vi "spring.vi"(7 "action (set itemstrings)":T1=enum."set itemstrings", 8 "error in (no error)":errorcluster, 9 "indentation/item symbols/colors in":i32[](array[numeric]), 10 "item strings in":string[][](array[string]), 11 "tree RefNum in":refnum<vi>) -> (0 "error out":errorcluster, 1 "item symbols/colors out":i32[](array[numeric]), 2 "item strings out":string[][](array[string]), 3 "dup tree RefNum":refnum<vi>)   [LabVIEW 2014]
uses:
  <userlib>/MSC-Tree/SW Code/Tree -string-/sub VIs/spring action.ctl
  <userlib>/MSC-Tree/SW Code/Tree -string-/sub VIs/spring - node data.ctl
panel:
  # "If you get error 16,\nthe number of columns\nin the input and tree\ndoes not match."
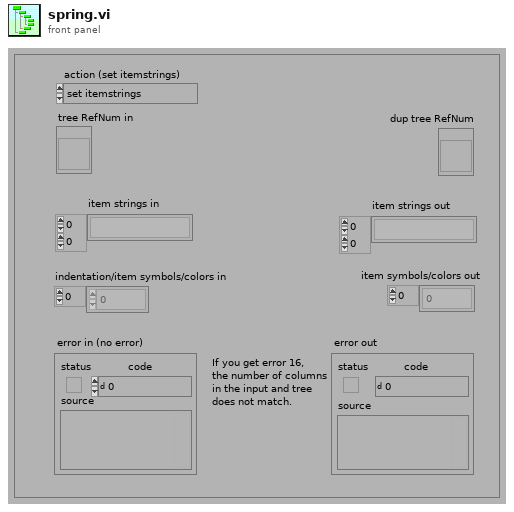
[diagram p1: front panel]
types:
  T1 = typedef "spring action.ctl" = enum16{"_init", "_add tree", "set itemstrings", "set fg colors", "set bg colors", "set symbols", "get tags", "get itemstrings", "get fg colors", "get bg colors", "get symbols", "empty tree", "update from tree"}
  T2 = typedef "spring - node data.ctl" = cluster{"tag":string, "indentation":i32, "itemstrings":string[], "fg color":i32, "bg color":i32, "symbol":i32}
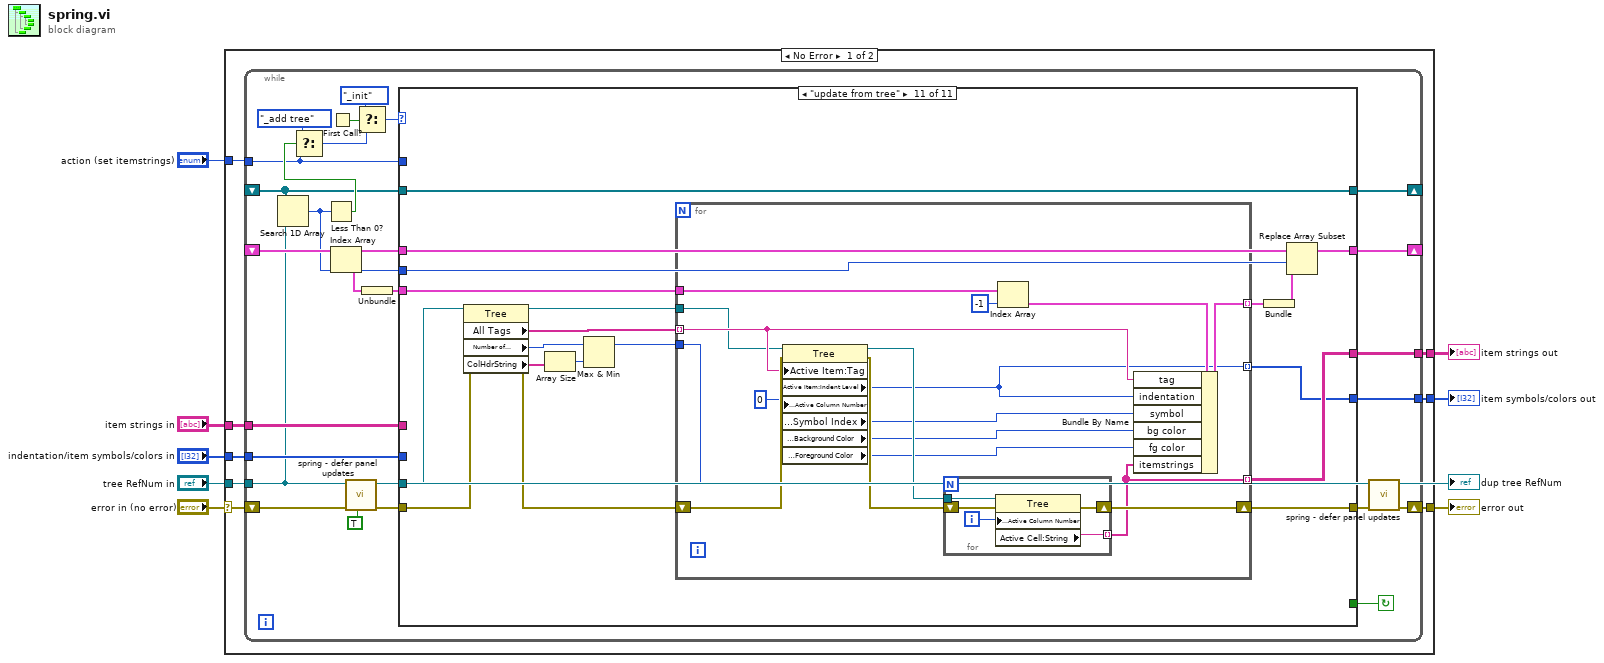
[diagram p0: block diagram]
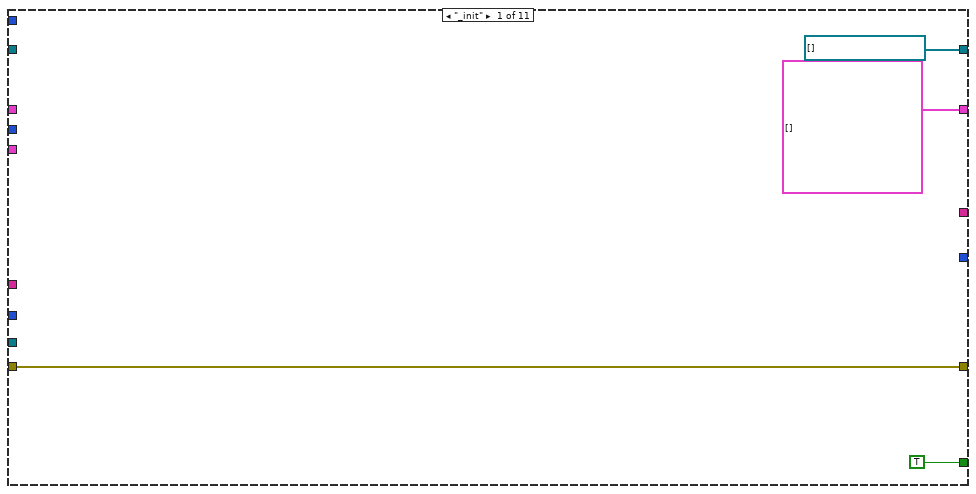
[diagram p2: hidden frame]
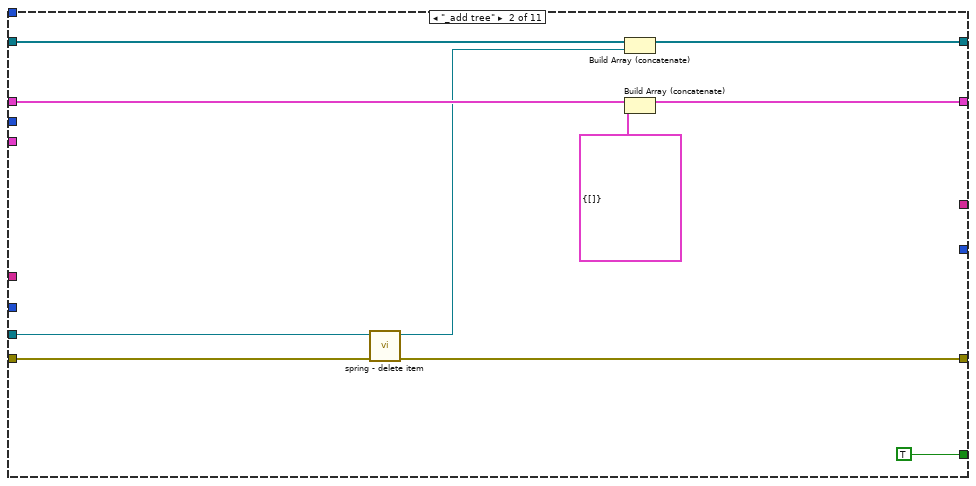
[diagram p3: hidden frame]
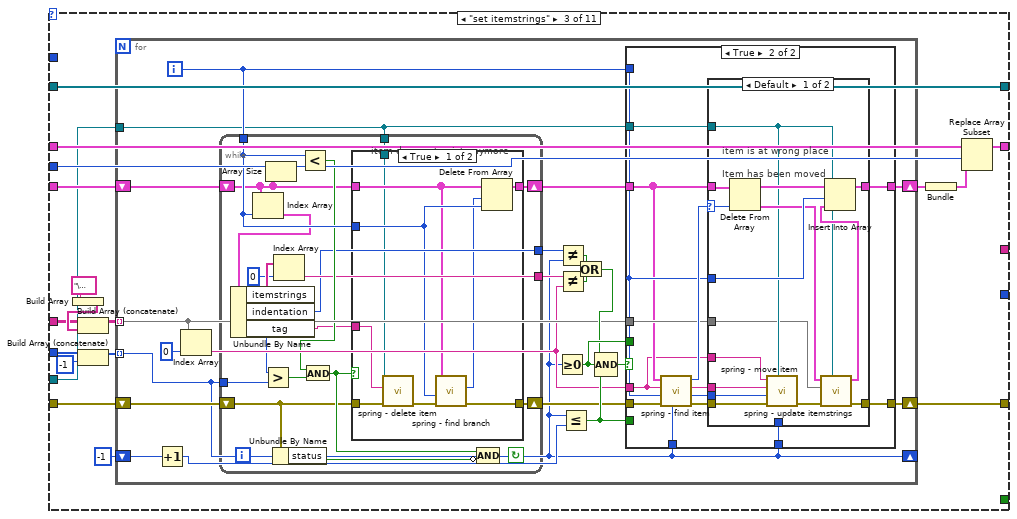
[diagram p4: hidden frame]
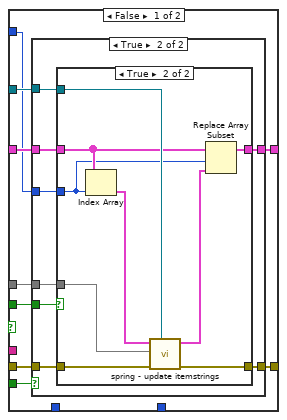
[diagram p6: hidden frame]
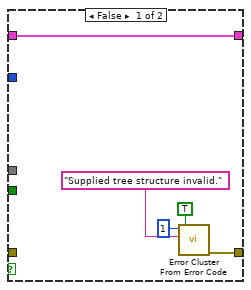
[diagram p7: hidden frame]
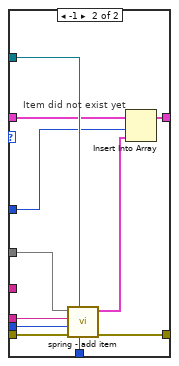
[diagram p9: hidden frame]
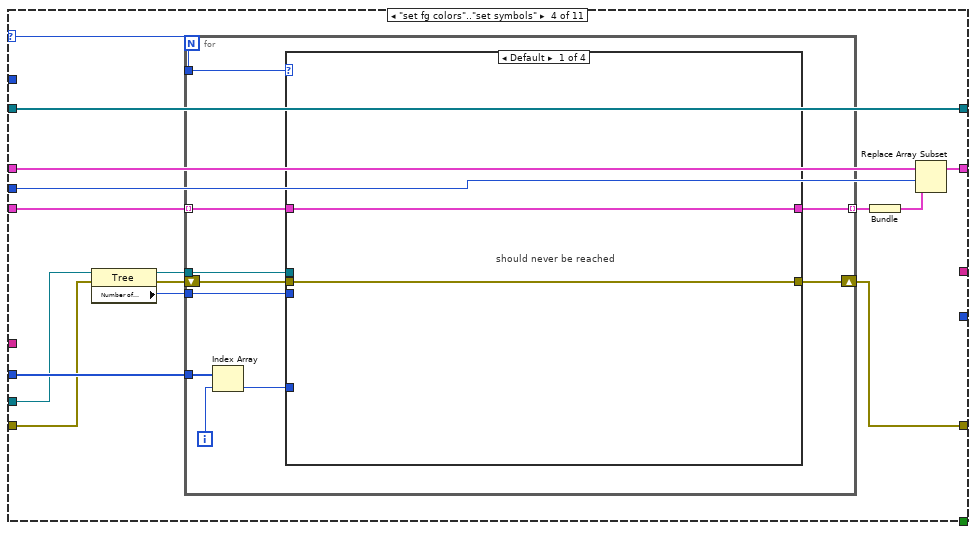
[diagram p10: hidden frame]
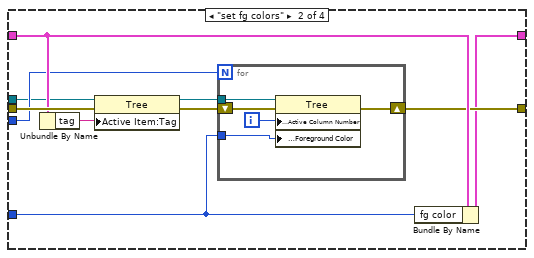
[diagram p11: hidden frame]
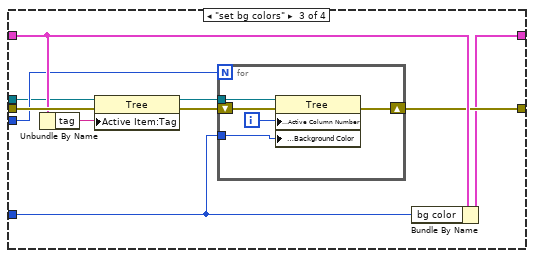
[diagram p12: hidden frame]
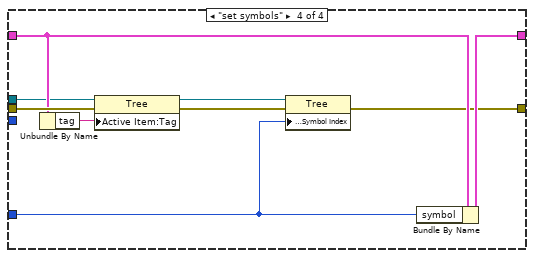
[diagram p13: hidden frame]
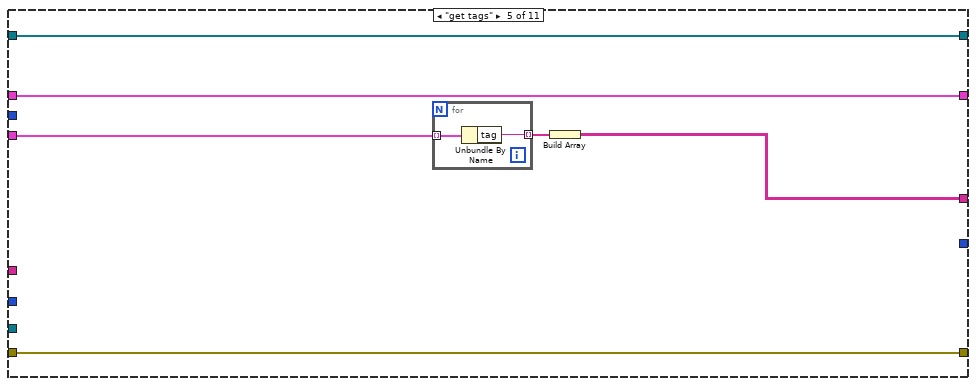
[diagram p14: hidden frame]
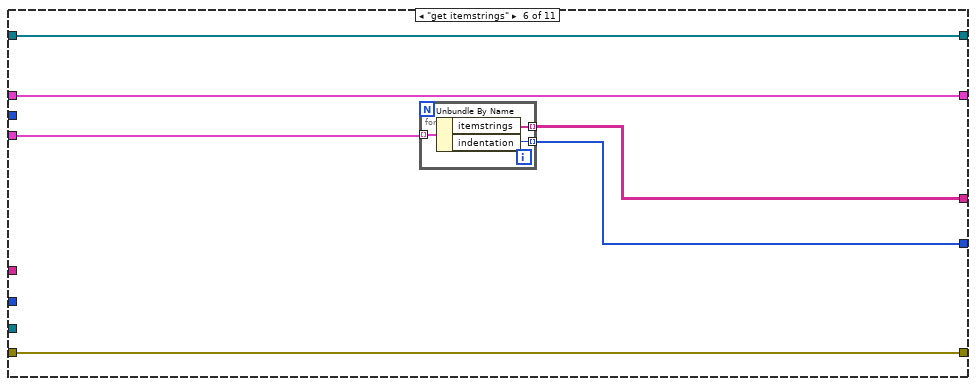
[diagram p15: hidden frame]
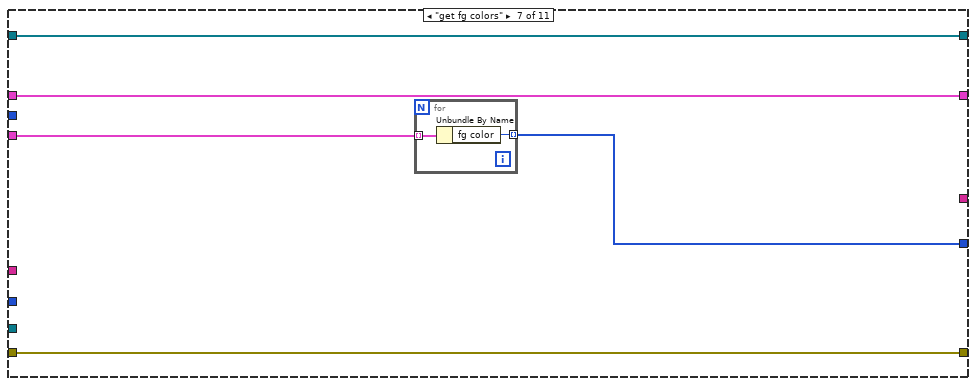
[diagram p16: hidden frame]
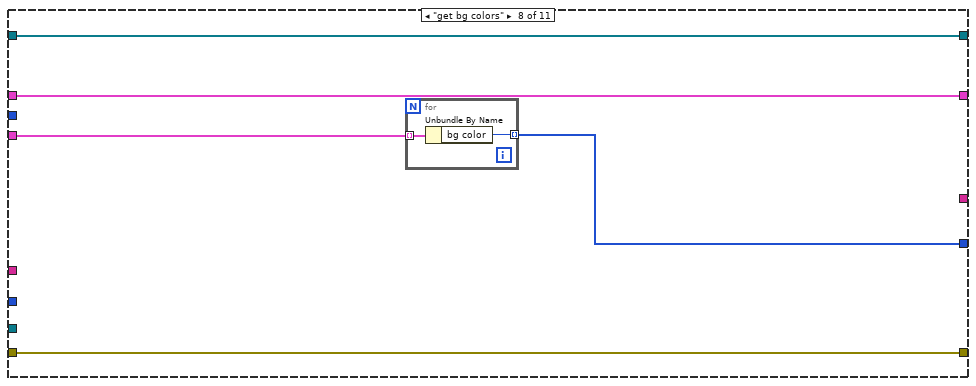
[diagram p17: hidden frame]
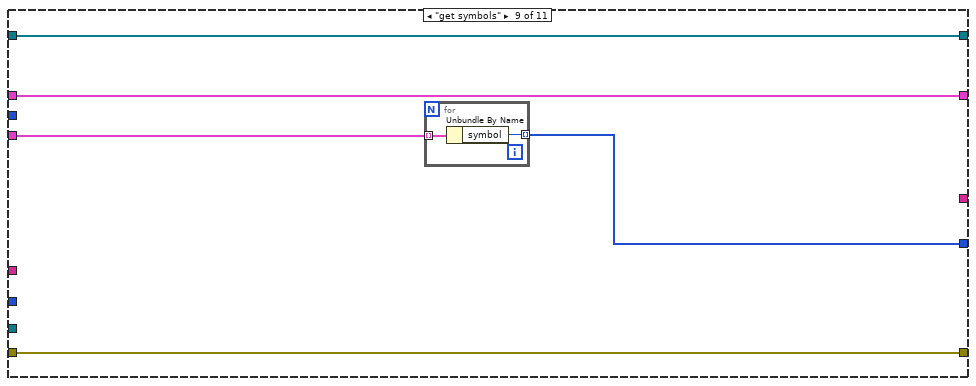
[diagram p18: hidden frame]
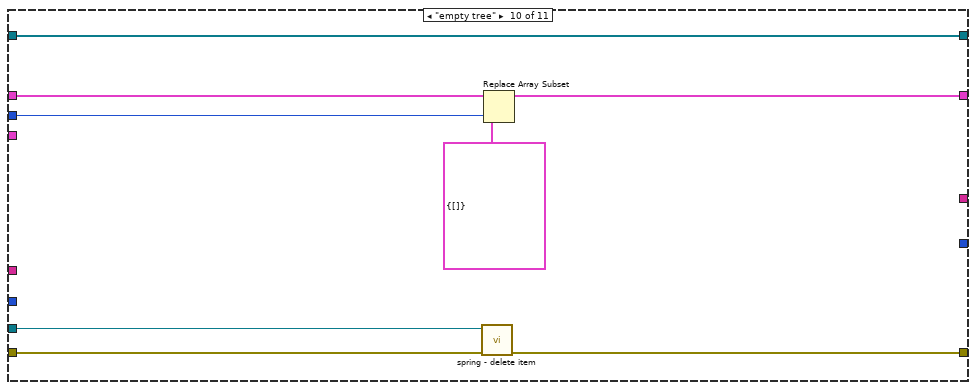
[diagram p19: hidden frame]
diagram:
  n1 = case shown="No Error" "error in (no error)" {
    selector: "error in (no error)" -> [w15 w353]
    tunnel: "tree RefNum in" -> [w16 _]
    tunnel: [w14 w353] -> w4
    tunnel: "item strings in" -> [w13 _]
    tunnel: "action (set itemstrings)" -> [w12 _]
    tunnel: [w11 _] -> w3
    tunnel: "indentation/item symbols/colors in" -> [w10 _]
    tunnel: [w9 _] -> w6
    frame No Error {
      n2 = while {
        tunnel: w16 -> [w19]
        shift-right: [w37] -> _
        shift-left: _ -> [w36]
        shift-right: [w23] -> w14
        shift-left: w15 -> [w22]
        tunnel: w13 -> [w35]
        shift-right: [w33] -> _
        shift-left: _ -> [w32]
        tunnel: [w29] -> w11
        tunnel: w10 -> [w26]
        tunnel: [w25] -> w9
        tunnel: w12 -> [w17]
        stop <- w34 continue-if-true
        n3 = Search 1D Array(1D array=w36, element=w19) -> (index of element=w30:i32)  [unwired: 1 out]
        n4 = Less Than 0?(x=w30) -> (x < 0?=w40:bool)
        n5 = Select(t=spring_action."_add tree" ("action"), s=w40, f=w17) -> (s? t:f=w42:T1)
        n6 = First Call?() -> (First Call?: T/F=w41:bool)
        n7 = Index Array(array=w32, index=w30) -> (element=w28:cluster{T2[]})
        n8 = call <userlib>:"spring - defer panel updates.vi"("defer panelUpdates (F)"=TRUE ("enable panel updates"), "error in (no error)"=w22, "RefNum in"=w19) -> ("error out"=w20:errorcluster, "dup RefNum"=w18:refnum<vi>)  [unwired: 2 in, 5 out]
        n9 = Select(t=spring_action."_init" ("action"), s=w41, f=w42) -> (s? t:f=w39:T1)
        n10 = Unbundle(w28) -> (w27:T2[])
        n11 = case shown="\"update from tree\"" w39 {
          selector: w39 -> [_ _ _ w206 _ _ _ _ _ _ _]
          tunnel: w20 -> [w45 w51 w58 w202 w269 w274 w285 w292 w299 w309 w321]
          tunnel: [w45 w50 w59 w200 w269 w274 w285 w292 w299 w308 w322] -> w24
          tunnel: w17 -> [_ _ _ _ _ _ _ _ _ _ _]
          tunnel: [refnum<vi>[] [] ("initialized array") w56 w74 w214 w270 w278 w286 w293 w300 w305 w330] -> w37
          tunnel: w36 -> [_ w55 w74 w214 w270 w278 w286 w293 w300 w305 w330]
          tunnel: w35 -> [_ _ w60 _ _ _ _ _ _ _ _]
          tunnel: [TRUE TRUE _ _ _ _ _ _ _ _ _] -> w34
          tunnel: w30 -> [_ _ w71 w211 _ _ _ _ _ w306 w328]
          tunnel: w32 -> [_ w52 w72 w212 w271 w279 w287 w294 w301 w311 w329]
          tunnel: [cluster{T2[]}[] [] ("initialized array") w54 w73 w213 w271 w279 w287 w294 w301 w310 w319] -> w33
          tunnel: [_ _ _ _ w267 w276 _ _ _ _ w324] -> w29
          tunnel: w27 -> [_ _ w65 w209 w268 w277 w284 w291 w298 _ w325]
          tunnel: w26 -> [_ _ w63 w203 _ _ _ _ _ _ _]
          tunnel: [_ _ _ _ _ w275 w283 w290 w297 _ w323] -> w25
          tunnel: w18 -> [_ w48 w57 w201 _ _ _ _ _ w307 w320]
          frame "_init" {
          }
          frame "_add tree" {
            n12 = call <userlib>:"spring - delete item.vi"("error in (no error)"=w51, "RefNum in"=w48) -> ("error out"=w50:errorcluster, "dup RefNum"=w49:refnum<vi>)  [unwired: 2 in, 6 out]
            n13 = Build Array (concatenate)(w55, w49) -> (w56:refnum<vi>[])
            n14 = Build Array (concatenate)(w52, cluster{T2[]} {[]} ("node data")) -> (w54:cluster{T2[]}[])
          }
          frame "set itemstrings" {
            n15 = Build Array("\u0000" ("String")) -> (w68:string[])
            n16 = Build Array (concatenate)(w60, w68) -> (w69:string[][])
            n17 = Build Array (concatenate)(w63, -1 ("disabled index (col)")) -> (w62:i32[])
            n18 = for {
              shift-right: [w92] -> w59
              shift-left: w58 -> [w84]
              tunnel: w57 -> [w89]
              tunnel: w69 -> [w78] mode=indexing
              shift-right: [w96] -> w64
              shift-left: w65 -> [w95]
              shift-right: [w76] -> _
              shift-left: -1 ("indentation") -> [w88]
              tunnel: w62 -> [w76] mode=indexing
              i -> [w91]
              n19 = Increment(x=w88) -> (x+1=w87:i32)
              n20 = Index Array(array=w78, index=0) -> (element=w77:string)
              n21 = while {
                tunnel: w89 -> [w113]
                shift-right: [w115] -> w94
                shift-left: w95 -> [w107]
                shift-right: [w114] -> w83
                shift-left: w84 -> [w98]
                tunnel: w91 -> [w110]
                tunnel: [w103] -> w93
                tunnel: w76 -> [w111]
                tunnel: [w102] -> w79
                stop <- w99 continue-if-true
                n22 = Index Array(array=w107, index=w110) -> (element=w106:T2)
                n23 = Unbundle By Name(w106) -> ("itemstrings"=w105:string[], "indentation"=w102:i32, "tag"=w101:string)
                n24 = Greater?(x=w102, y=w111) -> (0:w112:bool)
                n25 = Array Size(array=w107) -> (size(s)=w109:i32)
                n26 = Unbundle By Name(w98) -> ("status"=w97:bool)
                n27 = Index Array(array=w105, index=0) -> (element=w103:string)
                n28 = Less?(x=w110, y=w109) -> (x < y?=w108:bool)
                n29 = And(x=w108, y=w112) -> (x .and. y?=w100:bool)
                n30 = case shown="True" w100 {
                  tunnel: w107 -> [w118 w126]
                  tunnel: w98 -> [w124 w125]
                  tunnel: [w122 w125] -> w114
                  tunnel: w113 -> [w117 _]
                  tunnel: [w121 w126] -> w115
                  tunnel: w110 -> [w120 _]
                  tunnel: w101 -> [w116 _]
                  frame True {
                    # "item does not exist anymore"
                    n31 = call <userlib>:"spring - delete item.vi"("error in (no error)"=w124, "Tag (\"\" all)"=w116, "RefNum in"=w117) -> ("error out"=w123:errorcluster)  [unwired: 1 in, 7 out]
                    n32 = call <userlib>:"spring - find branch.vi"("error in (no error)"=w123, "branch index"=w120, "tree data"=w118) -> ("error out"=w122:errorcluster, "branch size"=w119:i32)  [unwired: 1 in, 6 out]
                    n33 = Delete From Array(array=w118, length=w119, index=w120) -> (array with subset deleted=w121:T2[])  [unwired: 1 out]
                  }
                  frame False {
                  }
                }
                n34 = Compound Arithmetic op=AND(w100, invert w97) -> (w99:bool)
              }
              n35 = Greater Or Equal To 0?(x=w76) -> (x >= 0?=w85:bool)
              n36 = Not Equal?(x=w79, y=w76) -> (x != y?=w80:bool)
              n37 = Not Equal?(x=w93, y=w77) -> (x != y?=w82:bool)
              n38 = Less Or Equal?(x=w76, y=w87) -> (x <= y?=w86:bool)
              n39 = Or(x=w80, y=w82) -> (x .or. y?=w81:bool)
              n40 = Compound Arithmetic op=AND(w81, w85, w86) -> (w90:bool)
              n41 = case shown="True" w90 {
                tunnel: w94 -> [w132 w166]
                tunnel: w83 -> [w134 w170]
                tunnel: [w133 w173] -> w92
                tunnel: w89 -> [w130 w172]
                tunnel: [w131 w171] -> w96
                tunnel: w91 -> [w127 w168]
                tunnel: w78 -> [w129 w167]
                tunnel: w86 -> [w135 _]
                tunnel: w77 -> [_ w165]
                tunnel: w85 -> [w128 _]
                tunnel: w76 -> [_ w164]
                tunnel: w76 -> [_ w160]
                frame False {
                  n42 = case shown="True" w135 {
                    tunnel: w134 -> [_ w148]
                    tunnel: [w139 w146] -> w133
                    tunnel: w132 -> [w140 w147]
                    tunnel: [w140 w144] -> w131
                    tunnel: w130 -> [_ w145]
                    tunnel: w129 -> [_ w143]
                    tunnel: w128 -> [_ w142]
                    tunnel: w127 -> [_ w141]
                    frame False {
                      n43 = call <vilib>:"Error Cluster From Error Code.vi"("show call chain? (False)"=TRUE, "error message (\"\")"="Supplied tree structure invalid." ("format string"), "error code (0)"=1) -> ("error out"=w139:errorcluster)  [unwired: 1 in, 5 out]
                    }
                    frame True {
                      n44 = case shown="True" w142 {
                        tunnel: w148 -> [w149 w154]
                        tunnel: w147 -> [w150 w153]
                        tunnel: [w149 w159] -> w146
                        tunnel: w145 -> [_ w157]
                        tunnel: [w150 w156] -> w144
                        tunnel: w143 -> [_ w155]
                        tunnel: w141 -> [_ w151]
                        frame False {
                          # "We've encountered the\ndummy \\00 item that was prepended\nat the start."
                        }
                        frame True {
                          n45 = Index Array(array=w153, index=w151) -> (element=w152:T2)
                          n46 = call <userlib>:"spring - update itemstrings.vi"("tree ref"=w157, "error in (no error)"=w154, "itemstrings"=w155, "node data"=w152) -> ("error out"=w159:errorcluster, "node data out"=w158:T2)  [unwired: 6 out]
                          n47 = Replace Array Subset(array=w153, new element=w158, index=w151) -> (w156:T2[])
                        }
                      }
                    }
                  }
                }
                frame True {
                  n48 = call <userlib>:"spring - find item.vi"("indentation"=w164, "error in (no error)"=w170, "item index"=w168, "primary itemstring to be found"=w165, "tree data"=w166) -> ("error out"=w161:errorcluster, "son# (0=first)"=w163:i32, "parent tag"=w162:string, "moved item's index"=w169:i32)  [unwired: 3 out]
                  n49 = case shown="Default" w169 {
                    selector: w169 -> [w184 _]
                    tunnel: w166 -> [w187 w196]
                    tunnel: w161 -> [w188 w194]
                    tunnel: [w181 w199] -> w173
                    tunnel: w172 -> [w177 w198]
                    tunnel: [w185 w197] -> w171
                    tunnel: w168 -> [w183 w195]
                    tunnel: w167 -> [w176 w189]
                    tunnel: w165 -> [w178 _]
                    tunnel: w163 -> [w175 w192]
                    tunnel: w162 -> [w174 w190]
                    tunnel: w160 -> [_ w191]
                    frame Default {
                      # "Item has been moved"
                      # "item is at wrong place"
                      n50 = Delete From Array(array=w187, index=w184) -> (deleted portion=w180:T2, array with subset deleted=w186:T2[])  [unwired: 1 in]
                      n51 = call <userlib>:"spring - move item.vi"("tree ref"=w177, "error in (no error)"=w188, "position (0=just below parent etc.)"=w175, "parent tag"=w174, "tag"=w178) -> ("error out"=w182:errorcluster)  [unwired: 6 out]
                      n52 = call <userlib>:"spring - update itemstrings.vi"("tree ref"=w177, "error in (no error)"=w182, "itemstrings"=w176, "node data"=w180) -> ("error out"=w181:errorcluster, "node data out"=w179:T2)  [unwired: 6 out]
                      n53 = Insert Into Array(array=w186, index=w183, new element=w179) -> (w185:T2[])
                    }
                    frame -1 {
                      # "Item did not exist yet"
                      n54 = call <userlib>:"spring - add item.vi"("new indentation"=w191, "tree ref"=w198, "error in (no error)"=w194, "position (0=just below parent etc.)"=w192, "parent tag"=w190, "itemstrings"=w189) -> ("error out"=w199:errorcluster, "node data out"=w193:T2)  [unwired: 4 out]
                      n55 = Insert Into Array(array=w196, index=w195, new element=w193) -> (w197:T2[])
                    }
                  }
                }
              }
            }
            n56 = Bundle(w64) -> (w70:cluster{T2[]})  [unwired: 1 in]
            n57 = Replace Array Subset(array=w72, new element=w70, index=w71) -> (w73:cluster{T2[]}[])
          }
          frame "set fg colors".."set symbols" {
            n58 = property on="Property Node" class="Tree"(reference=w201, error in=w202) -> (reference out=w204:refnum<vi>, error out=w207:errorcluster, "Number of Columns"=w208:u32)
            n59 = for {
              shift-right: [w221] -> w200
              shift-left: w207 -> [w224]
              tunnel: w204 -> [w218]
              tunnel: w209 -> [w223] mode=indexing
              tunnel: w208 -> [w222]
              tunnel: w206 -> [w219]
              tunnel: [w220] -> w205 mode=indexing
              tunnel: w203 -> [w217]
              i -> [w216]
              n60 = Index Array(array=w217, index=w216) -> (element=w215:i32)
              n61 = case shown="Default" w219 {
                tunnel: w224 -> [w226 w236 w251 w265]
                tunnel: w223 -> [w225 w234 w249 w264]
                tunnel: w222 -> [_ w233 w248 _]
                tunnel: [w226 w232 w247 w258] -> w221
                tunnel: [w225 w231 w246 w263] -> w220
                tunnel: w215 -> [_ w229 w244 w257]
                tunnel: w218 -> [_ w227 w242 w261]
                frame Default {
                  # "should never be reached"
                }
                frame "set fg colors" {
                  n62 = Unbundle By Name(w234) -> ("tag"=w230:string)
                  n63 = property on="Property Node" class="Tree"(reference=w227, error in=w236, "Active Item:Tag"=w230) -> (reference out=w228:refnum<vi>, error out=w235:errorcluster)
                  n64 = for {
                    N: w233 -> [_]
                    shift-right: [w239] -> w232
                    shift-left: w235 -> [w241]
                    tunnel: w229 -> [w238]
                    tunnel: w228 -> [w237]
                    i -> [w240]
                    n65 = property on="Property Node" class="Tree"(reference=w237, error in=w241, "Active Cell:Active Column Number"=w240, "Active Cell:Foreground Color"=w238) -> (error out=w239:errorcluster)  [unwired: 1 out]
                  }
                  n66 = Bundle By Name(cluster=w234, "fg color"=w229) -> (w231:T2)
                }
                frame "set bg colors" {
                  n67 = Unbundle By Name(w249) -> ("tag"=w245:string)
                  n68 = property on="Property Node" class="Tree"(reference=w242, error in=w251, "Active Item:Tag"=w245) -> (reference out=w243:refnum<vi>, error out=w250:errorcluster)
                  n69 = for {
                    N: w248 -> [_]
                    shift-right: [w254] -> w247
                    shift-left: w250 -> [w256]
                    tunnel: w244 -> [w253]
                    tunnel: w243 -> [w252]
                    i -> [w255]
                    n70 = property on="Property Node" class="Tree"(reference=w252, error in=w256, "Active Cell:Active Column Number"=w255, "Active Cell:Background Color"=w253) -> (error out=w254:errorcluster)  [unwired: 1 out]
                  }
                  n71 = Bundle By Name(cluster=w249, "bg color"=w244) -> (w246:T2)
                }
                frame "set symbols" {
                  n72 = Unbundle By Name(w264) -> ("tag"=w262:string)
                  n73 = property on="Property Node" class="Tree"(reference=w261, error in=w265, "Active Item:Tag"=w262) -> (reference out=w260:refnum<vi>, error out=w259:errorcluster)
                  n74 = property on="Property Node" class="Tree"(reference=w260, error in=w259, "Active Item:Symbol Index"=w257) -> (error out=w258:errorcluster)  [unwired: 1 out]
                  n75 = Bundle By Name(cluster=w264, "symbol"=w257) -> (w263:T2)
                }
              }
            }
            n76 = Bundle(w205) -> (w210:cluster{T2[]})  [unwired: 1 in]
            n77 = Replace Array Subset(array=w212, new element=w210, index=w211) -> (w213:cluster{T2[]}[])
          }
          frame "get tags" {
            n78 = for {
              tunnel: w268 -> [w273] mode=indexing
              tunnel: [w272] -> w266 mode=indexing
              n79 = Unbundle By Name(w273) -> ("tag"=w272:string)
            }
            n80 = Build Array(w266) -> (w267:string[][])
          }
          frame "get itemstrings" {
            n81 = for {
              tunnel: w277 -> [w282] mode=indexing
              tunnel: [w281] -> w276 mode=indexing
              tunnel: [w280] -> w275 mode=indexing
              n82 = Unbundle By Name(w282) -> ("itemstrings"=w281:string[], "indentation"=w280:i32)
            }
          }
          frame "get fg colors" {
            n83 = for {
              tunnel: w284 -> [w289] mode=indexing
              tunnel: [w288] -> w283 mode=indexing
              n84 = Unbundle By Name(w289) -> ("fg color"=w288:i32)
            }
          }
          frame "get bg colors" {
            n85 = for {
              tunnel: w291 -> [w296] mode=indexing
              tunnel: [w295] -> w290 mode=indexing
              n86 = Unbundle By Name(w296) -> ("bg color"=w295:i32)
            }
          }
          frame "get symbols" {
            n87 = for {
              tunnel: w298 -> [w303] mode=indexing
              tunnel: [w302] -> w297 mode=indexing
              n88 = Unbundle By Name(w303) -> ("symbol"=w302:i32)
            }
          }
          frame "empty tree" {
            n89 = call <userlib>:"spring - delete item.vi"("error in (no error)"=w309, "RefNum in"=w307) -> ("error out"=w308:errorcluster)  [unwired: 2 in, 7 out]
            n90 = Replace Array Subset(array=w311, new element=cluster{T2[]} {[]} ("node data"), index=w306) -> (w310:cluster{T2[]}[])
          }
          frame "update from tree" {
            n91 = property on="Property Node" class="Tree"(reference=w320, error in=w321) -> (reference out=w316:refnum<vi>, error out=w318:errorcluster, "All Tags"=w317:string[], "Number of Columns"=w313:u32, "ColHdrString"=w315:string[])
            n92 = Array Size(array=w315) -> (size(s)=w314:i32)
            n93 = Max & Min(x=w313, y=w314) -> (max(x,y)=w312:u32)  [unwired: 1 out]
            n94 = for {
              shift-right: [w343] -> w322
              shift-left: w318 -> [w344]
              tunnel: w317 -> [w334] mode=indexing
              tunnel: w312 -> [w347]
              tunnel: [w339] -> w326 mode=indexing
              tunnel: w325 -> [w341]
              tunnel: [w333] -> w324 mode=indexing
              tunnel: [w332] -> w323 mode=indexing
              tunnel: w316 -> [w331]
              (unwired) 0 ("index")
              n95 = property on="Property Node" class="Tree"(reference=w331, error in=w344, "Active Item:Tag"=w334, "Active Cell:Active Column Number"=0 ("Active Cell Properties:Active Column Number")) -> (reference out=w346:refnum<vi>, error out=w345:errorcluster, "Active Item:Indent Level"=w332:i32, "Active Item:Symbol Index"=w338:i32, "Active Cell:Background Color"=w336:u32, "Active Cell:Foreground Color"=w335:u32)
              n96 = for {
                N: w347 -> [_]
                tunnel: w346 -> [w352]
                tunnel: [w348] -> w333 mode=indexing
                shift-right: [w349] -> w343
                shift-left: w345 -> [w350]
                i -> [w351]
                n97 = property on="Property Node" class="Tree"(reference=w352, error in=w350, "Active Cell:Active Column Number"=w351) -> (error out=w349:errorcluster, "Active Cell:String"=w348:string)  [unwired: 1 out]
              }
              n98 = Index Array(array=w341, index=-1) -> (element=w340:T2)
              n99 = Bundle By Name(cluster=w340, "tag"=w334, "indentation"=w332, "symbol"=w338, "bg color"=w336, "fg color"=w335, "itemstrings"=w333) -> (w339:T2)
            }
            n100 = Bundle(w326) -> (w327:cluster{T2[]})  [unwired: 1 in]
            n101 = Replace Array Subset(array=w329, new element=w327, index=w328) -> (w319:cluster{T2[]}[])
          }
        }
        n102 = call <userlib>:"spring - defer panel updates.vi"("error in (no error)"=w24, "RefNum in"=w18) -> ("error out"=w23:errorcluster)  [unwired: 3 in, 6 out]
      }
    }
    frame Error {
    }
  }
  "item symbols/colors out" <- w6
  "error out" <- w4
  "item strings out" <- w3
  "dup tree RefNum" <- "tree RefNum in"
